vi "nanocal_raw_file_manage_V1.vi"(7 "action":T2, 10 "list of lines IN":string[](array[string]), 11 "header IN":string) -> (0 "z (K/W)  OUT":cdb[](array[numeric]), 1 "f (Hz) OUT":dbl[](array[numeric]), 3 "header OUT":string)   [LabVIEW 2021]
uses:
  nanocal_raw_file_manage_fieldname_V1.ctl
  nanocal_raw_file_manage_action_V1.ctl
panel:
  out "test IN":string[][](array[string])
  out "Map":map{T1, i32}(c390)
  in  "Text Ring":u16(ring) items=["Time (s)", "Datapoint index", "Datapoint time (s)", "PHs (W)", "PHr (W)", "Ps,dc (W)", "Pr,dc (W)", "PHs,dc (W)", "PHr,dc (W)", "Ps,ac (W)", "Pr,ac (W)", "PHs/PHr", "Poffs (W)", "Ps total (W)", "Pr total (W)", "Ps-Pr total (W)", "Ps,offs (W)", "Ps,cond (W)", "Ps,net (W)", "Cs (J/K)", "Ks (W/K)", "Cr (J/K)", "Kr (W/K)", "Cdiff (J/K)", "Cs-Cr (J/K)", "Cdiff old style (J/K)", "Cr from S,diff (J/K)", "Cs from dT/dt (J/K)", "Ks,nom (W/K)", "Cs/T (J/K^2)", "Cr/T (J/K^2)", "Cdiff/T (J/K^2)", "(Cs-Cr)/T (J/K^2)", "Cdiff/T old style (J/K^2)", "Cr/T from S,diff (J/K^2)", "Ts (K)", "Tr (K)", "Tdiff from Rs,Rr", "Tdiff from Udiff (K)", "Ts,ac (K)", "Tr,ac (K)", "Tdiff,ac (K)", "Ts,ac driftcorr (K)", "Tr,ac driftcorr (K)", "Tr,ac from Ts,diff,ac (K)", "T target (K)", "Ts^2 (K^2)", "Tr^2 (K^2)", "Tcos/(P/K)", "Tsin/(P/K)", "H (T)", "T probe (K)", "Polar angle (deg)", "Azimuthal angle (deg)", "RHs (ohm)", "RHr (ohm)", "Rs (ohm)", "Rr (ohm)", "RHs,dc (ohm)", "RHr,dc (ohm)", "Rs,ac (ohm)", "Rr,ac (ohm)", "Roffs (ohm)", "f (Hz)", "f therm (Hz)", "omega (rad/s)", "Tan Phi S/diff", "Sin Phi", "Cos Phi", "f mix (Hz)", "tau (s)", "Phi Is (deg)", "Phi Us (deg)", "Phi Ir (deg)", "Phi Ur (deg)", "Phi Udiff (deg)", "Phi IHs (deg)", "Phi UHs (deg)", "Phi IHr (deg)", "Phi UHr (deg)", "Phi R from S,diff (deg)", "Phi Is 1st (deg)", "Phi Us 1st (deg)", "Phi Ir 1st (deg)", "Phi Ur 1st (deg)", "Phi Udiff 1st (deg)", "Phi Udiff, raw (deg)", "S phase (deg)", "R phase (deg)", "Diff phase (deg)", "Is,dc (A)", "Ir,dc (A)", "Us,dc (V)", "Ur,dc (V)", "Udiff,dc (V)", "IHs dc (A)", "UHs dc (V)", "IHr dc (A)", "UHr dc (V)", "Uoffs dc (V)", "Ioffs dc (A)", "Is,ac 1st (A)", "Ir,ac 1st (A)", "Us,ac 1st (V)", "Ur,ac 1st (V)", "Udiff,ac 1st (V)", "IHs (A)", "UHs (V)", "IHr (A)", "UHr (V)", "Is,ac (A)", "Ir,ac (A)", "Us,ac (V)", "Ur,ac (V)", "Udiff,ac (V)", "S out phase (deg)", "R out phase (deg)", "Hs ac out (Vrms)", "Hr ac out (Vrms)", "S Therm dc out (V)", "R Therm dc out (V)", "S Therm ac out (Vrms)", "R Therm ac out (Vrms)", "Offset dc out (V)", "Hs dc out (V)", "Hr dc out (V)", "Offset ac out (Vrms)", "1+Rs/RIs factor", "1+RIs/Rs factor", "Rs,scaled (ohm)", "Rr,scaled (ohm)", "R lead S (ohm)", "R lead R (ohm)", "|dlnR/dlnT| S", "|dlnR/dlnT| R", "dTs/dt (mK/s)", "dTr/dt (mK/s)", "Test"]
  in  "field names":T1
  out "Array":string[][](array[string])
  in  "String names":string
  in  "String numbers":string
  # "(* {62, (* Phs*) 4,(*Tac*)40, (*phase*)86} -- old file structure*)\n\na2 = rawdata[name]  // \n\n   map2[ {2 (* current to power*)   #[[62]],\n (* use Ts,ac   *) #[[40]]/#[[4]] Cos[ #[[86]]  Pi /180],  \n                            #[[40]]/#[[4]] Sin[ #[[86]]  Pi /180] \n\n} &] ;"
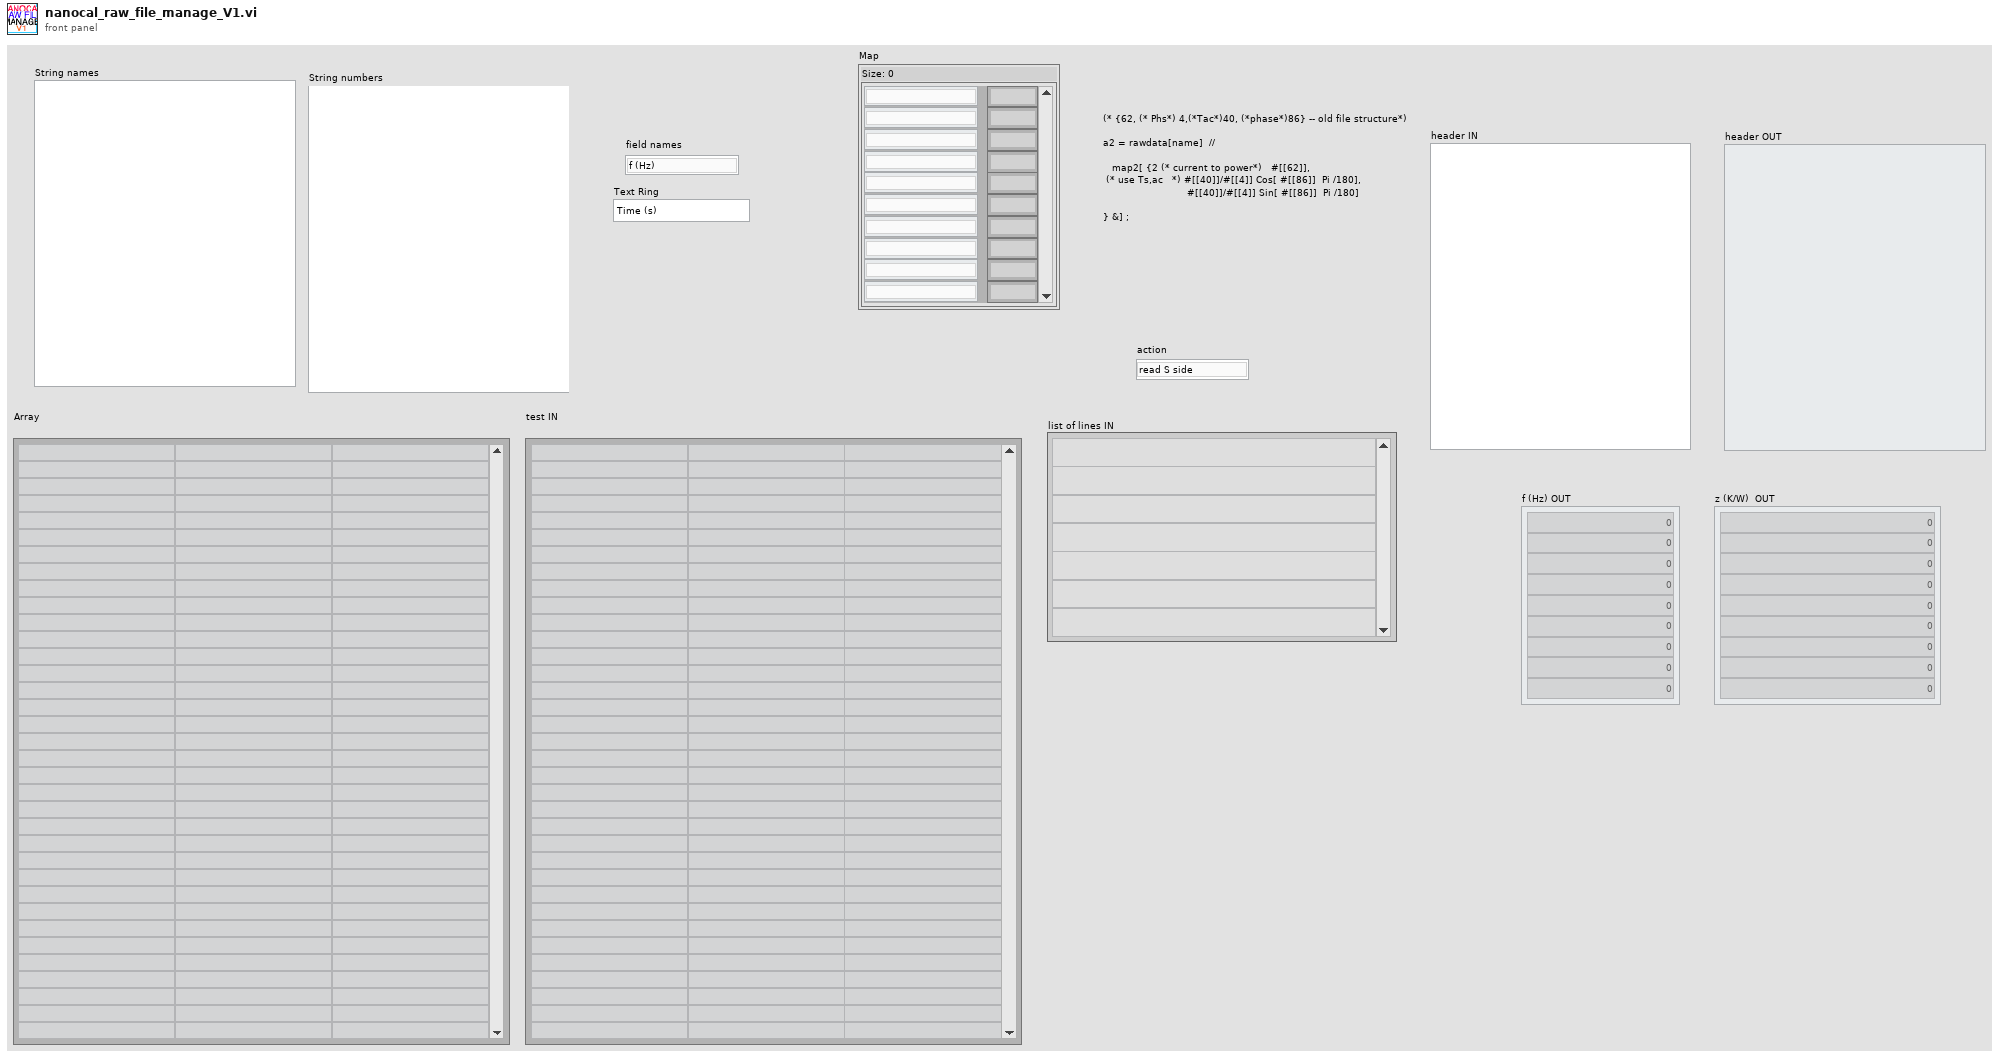
[diagram p1: front panel]
types:
  T1 = typedef "nanocal_raw_file_manage_fieldname_V1.ctl" = enum16{"f (Hz)", "S phase (deg)", "R phase (deg)", "Ts,ac (K)", "Tr,ac (K)", "PHs (W)", "PHr (W)", "Time (s)", "Tdiff,ac (K)", "Ts (K)", "Tr (K)"}
  T2 = typedef "nanocal_raw_file_manage_action_V1.ctl" = enum16{"read S side", "read R side", "read meta", "read_names"}
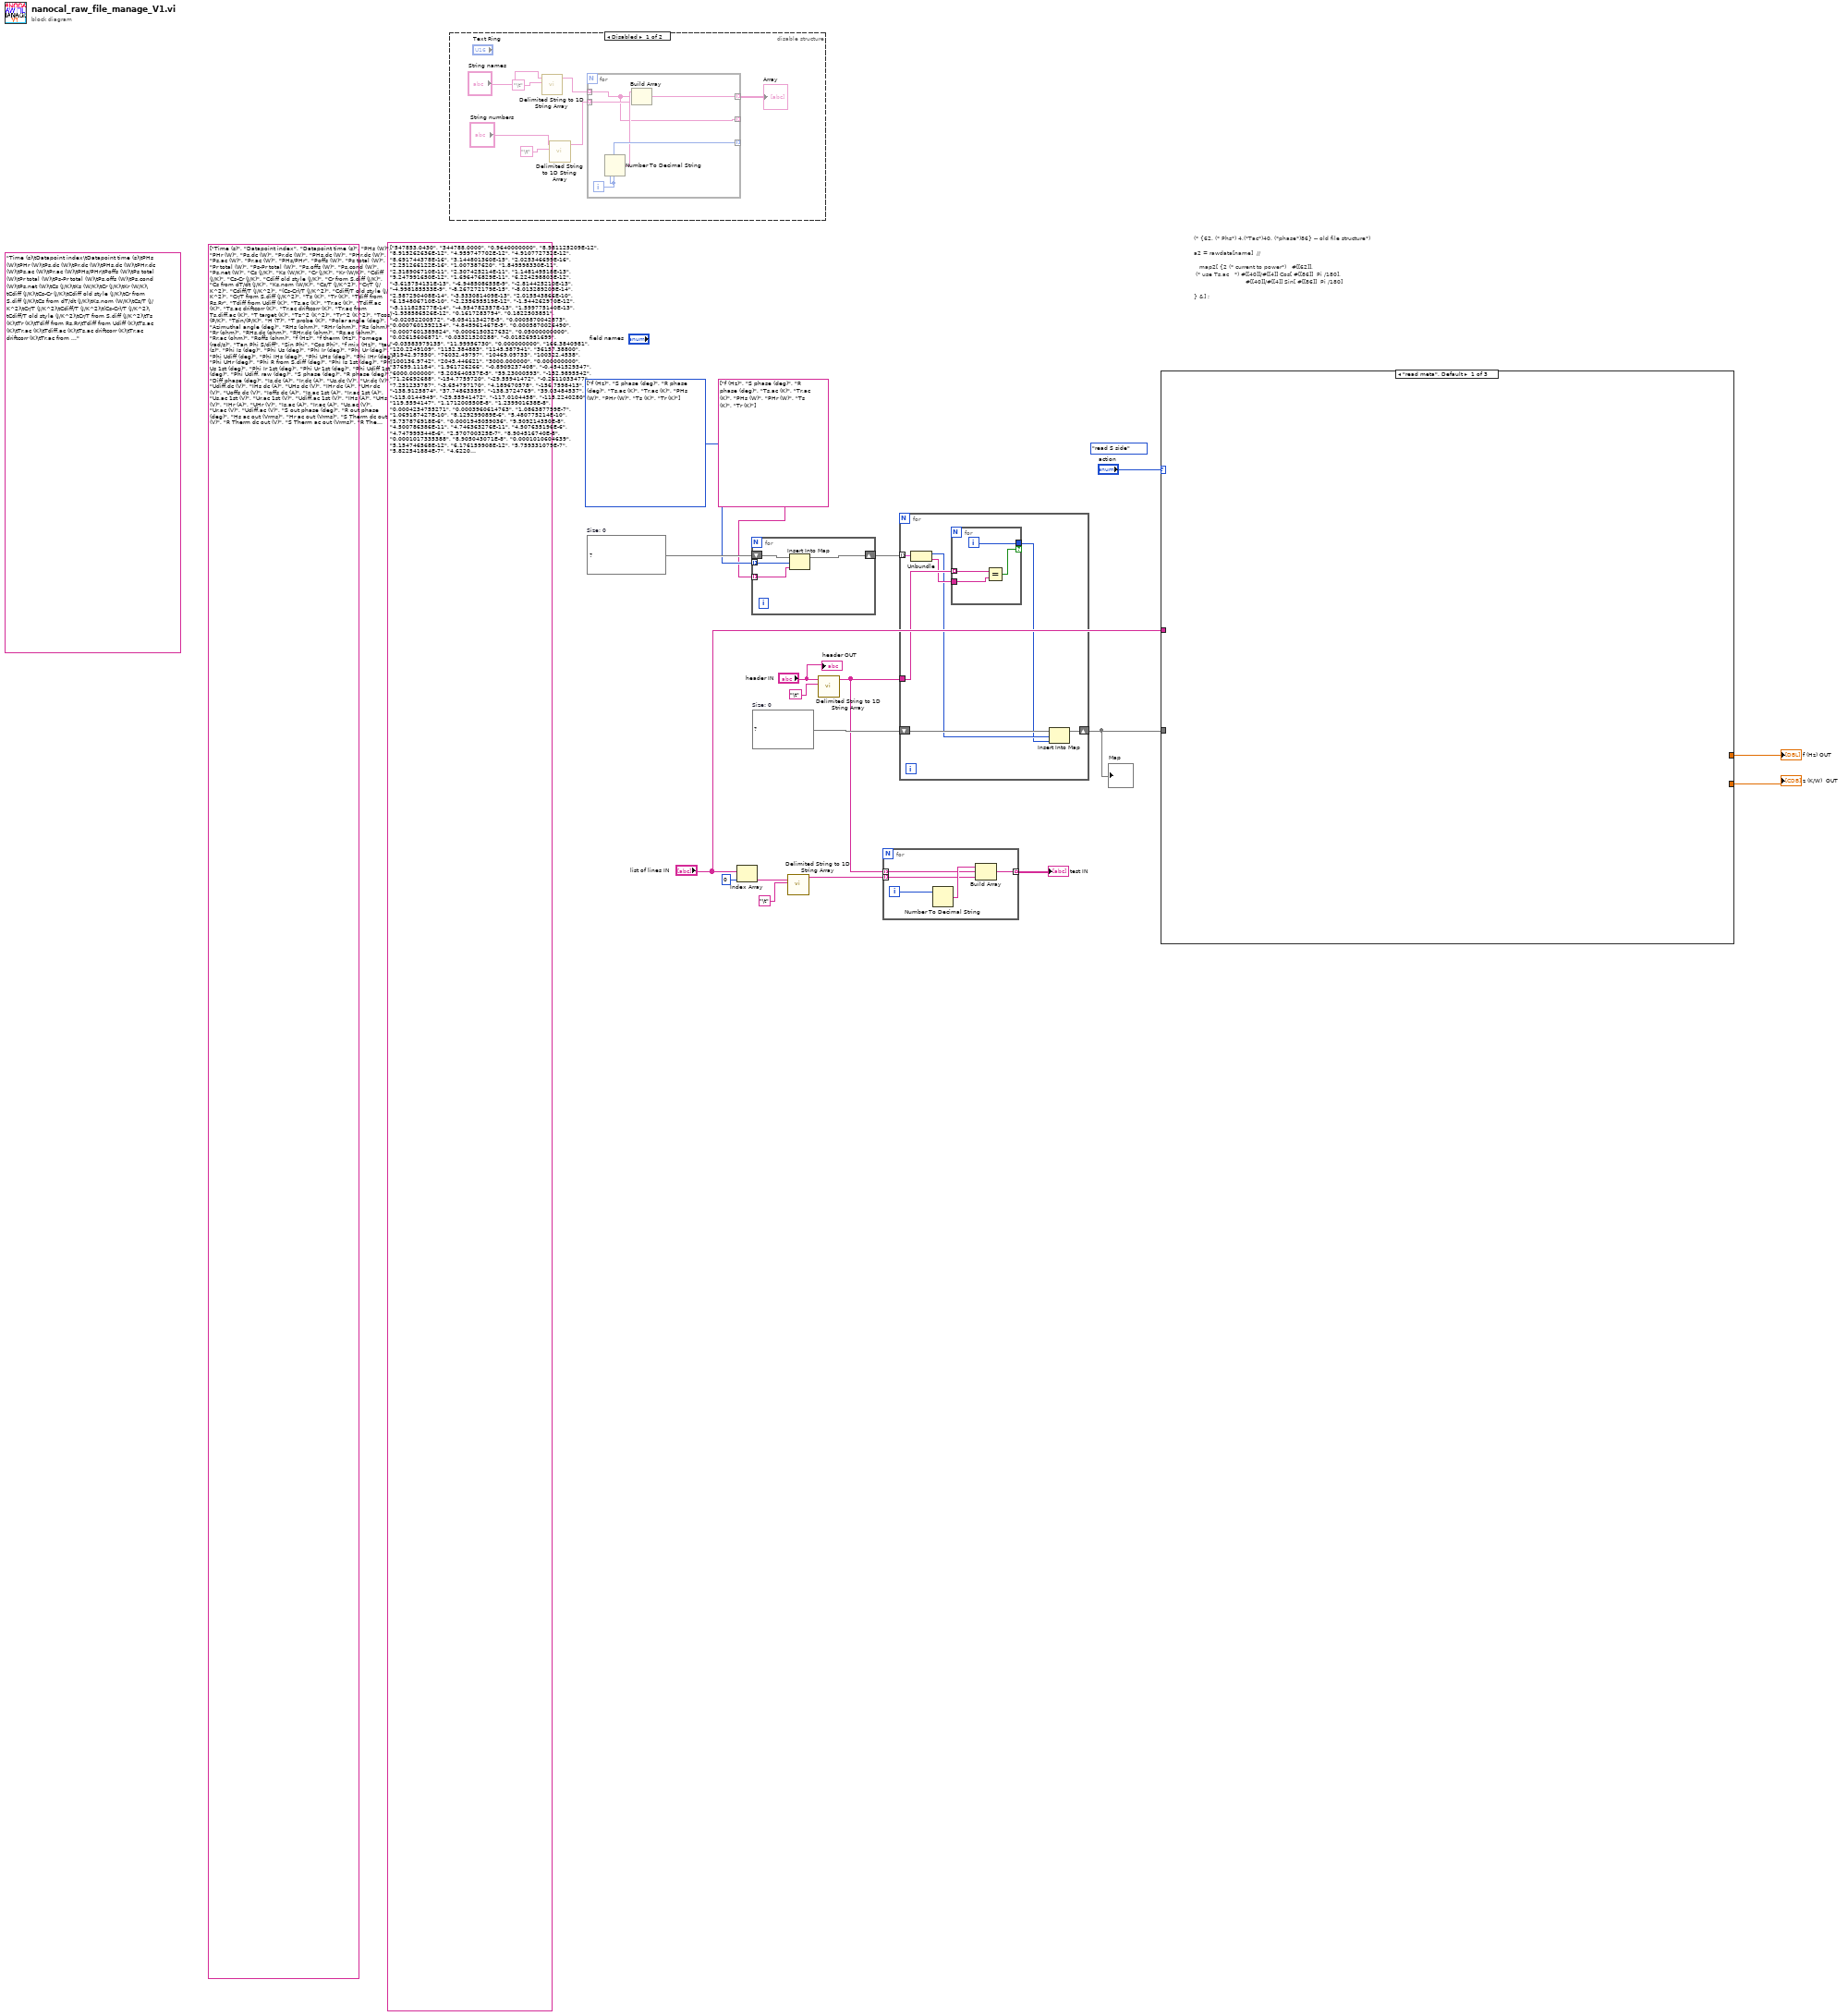
[diagram p0: block diagram]
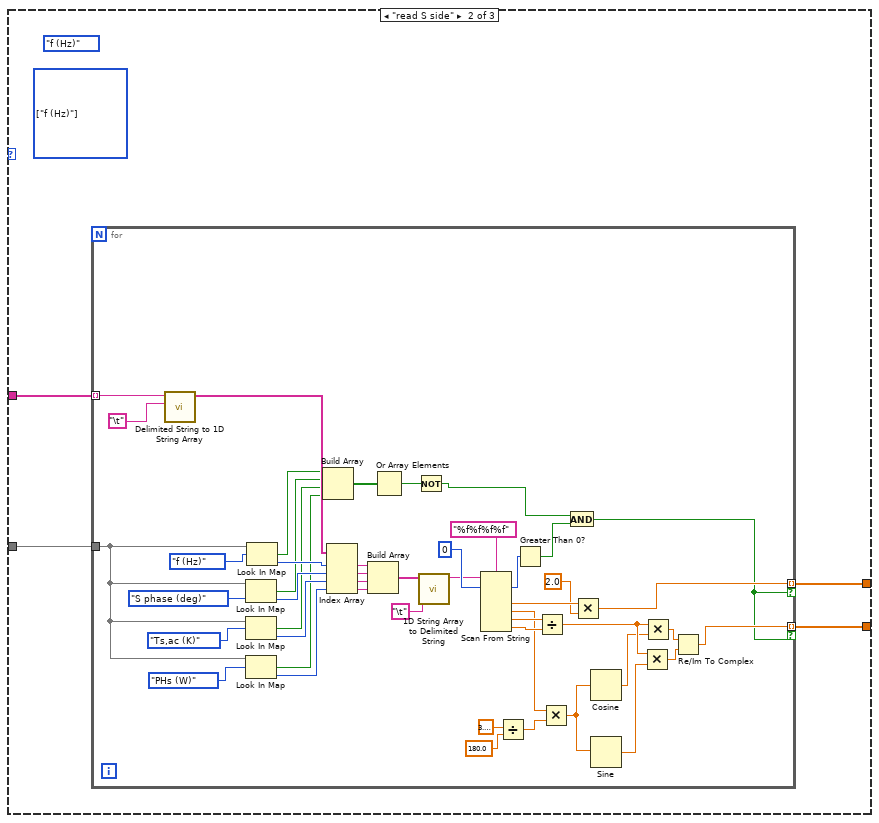
[diagram p3: hidden frame]
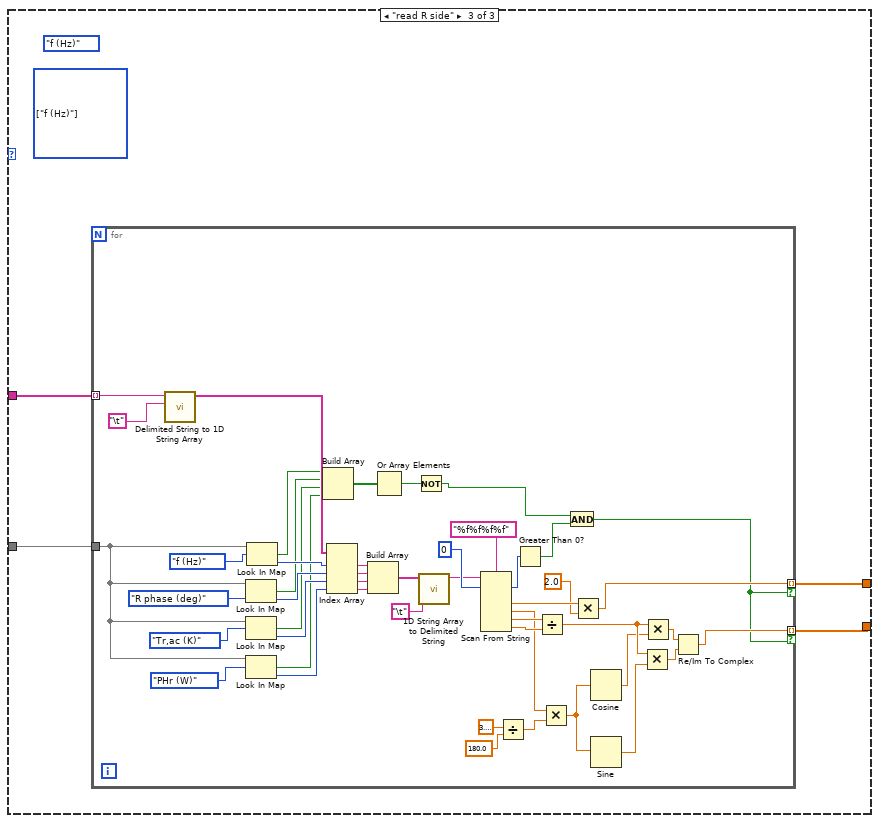
[diagram p4: hidden frame]
diagram:
  w13 = map{T1, i32} {}  # Size: 0
  w17 = map{T1, string} {}  # Size: 0
  w16 = T1[] [enum."f (Hz)", enum."S phase (deg)", enum."R phase (deg)", enum."Ts,ac (K)", enum."Tr,ac (K)", enum."PHs (W)", enum."PHr (W)", enum."Ts (K)", enum."Tr (K)"] items=["f (Hz)", "S phase (deg)", "R phase (deg)", "Ts,ac (K)", "Tr,ac (K)", "PHs (W)", "PHr (W)", "Time (s)", "Tdiff,ac (K)", "Ts (K)", "Tr (K)"]
  (unwired) nanocal_raw_file_manage_action_V1."read S side" ("Enum")
  (unwired) string[] ["547853.0430", "344788.0000", "0.9640000000", "8.981125209E-12", "8.915262636E-12", "4.959747702E-12", "4.910772732E-12", "8.691744378E-16", "3.144801360E-15", "2.025346699E-16", "2.251266122E-16", "1.007387620", "1.849598330E-11", "2.318906710E-11", "2.307425214E-11", "1.148149518E-13", "9.247991650E-12", "1.696476829E-11", "6.224298803E-12", "-3.615754131E-13", "-6.948508655E-9", "-2.814425210E-13", "-4.998185533E-9", "-8.267272179E-15", "-8.013289209E-14", "2.587290408E-14", "-3.533081409E-13", "2.015543866E-10", "6.154806710E-10", "-2.235695519E-12", "-1.544262970E-12", "-5.111825277E-14", "-4.954782357E-13", "1.599775140E-13", "-1.938586526E-12", "0.1617283794", "0.1822503851", "-0.02052200572", "-8.054113427E-5", "0.0005870042873", "0.0007601392134", "4.845961467E-5", "0.0005870026490", "0.0007601389824", "0.0006150327632", "0.05000000000", "0.02615606871", "0.03321520288", "-0.01826951699", "-0.03583979135", "11.99956730", "0.000000000", "166.3840981", "120.2249109", "1152.384883", "1145.587941", "36157.38800", "31942.97550", "76032.49797", "10469.09733", "100322.4538", "100136.9742", "2045.446621", "3000.000000", "0.000000000", "37699.11184", "1.961726266", "-0.8909237408", "-0.4541529347", "6000.000000", "5.203640537E-5", "59.23000593", "-152.9895542", "71.26692688", "-154.7759720", "-29.55941472", "-0.2611033477", "7.251233787", "-3.654797170", "4.189670578", "-156.7598413", "-138.9125874", "37.74863355", "-138.3724769", "39.03484537", "-115.0144949", "-29.55941472", "-117.0104458", "-115.2240280", "119.5594147", "1.171200550E-8", "1.239901638E-8", "0.0004234755271", "0.0003960614763", "1.086387799E-7", "1.069187427E-10", "8.129299089E-6", "5.480775214E-10", "5.737876918E-6", "0.0001945059036", "9.509214350E-8", "4.500786386E-11", "4.746363276E-11", "4.507635196E-6", "4.747999344E-6", "2.570700325E-7", "8.904516740E-8", "0.0001017335388", "8.905043071E-8", "0.0001010604639", "5.154746568E-12", "6.176159908E-12", "5.759331079E-7", "5.822541884E-7", "4.622022938E-8", "0.000000000", "0.000000000", "0.009030217479", "0.009030217479", "0.001382604241", "0.001487392001", "0.000000000", "0.000000000", "0.009530331008", "0.000000000", "0.000000000", "0.000000000", "1.361573880", "3.765686503", "36157.38800", "31942.97550", "-18107.21790", "-11982.49189", "0.7014008160", "0.6673683771", "0.03088148519", "0.004354902059", "1.234560000"] ("string array")
  (unwired) "Time (s)\tDatapoint index\tDatapoint time (s)\tPHs (W)\tPHr (W)\tPs,dc (W)\tPr,dc (W)\tPHs,dc (W)\tPHr,dc (W)\tPs,ac (W)\tPr,ac (W)\tPHs/PHr\tPoffs (W)\tPs total (W)\tPr total (W)\tPs-Pr total (W)\tPs,offs (W)\tPs,cond (W)\tPs,net (W)\tCs (J/K)\tKs (W/K)\tCr (J/K)\tKr (W/K)\tCdiff (J/K)\tCs-Cr (J/K)\tCdiff old style (J/K)\tCr from S,diff (J/K)\tCs from dT/dt (J/K)\tKs,nom (W/K)\tCs/T (J/K^2)\tCr/T (J/K^2)\tCdiff/T (J/K^2)\t(Cs-Cr)/T (J/K^2)\tCdiff/T old style (J/K^2)\tCr/T from S,diff (J/K^2)\tTs (K)\tTr (K)\tTdiff from Rs,Rr\tTdiff from Udiff (K)\tTs,ac (K)\tTr,ac (K)\tTdiff,ac (K)\tTs,ac driftcorr (K)\tTr,ac driftcorr (K)\tTr,ac from Ts,diff,ac (K)\tT target (K)\tTs^2 (K^2)\tTr^2 (K^2)\tTcos/(P/K)\tTsin/(P/K)\tH (T)\tT probe (K)\tPolar angle (deg)\tAzimuthal angle (deg)\tRHs (ohm)\tRHr (ohm)\tRs (ohm)\tRr (ohm)\tRHs,dc (ohm)\tRHr,dc (ohm)\tRs,ac (ohm)\tRr,ac (ohm)\tRoffs (ohm)\tf (Hz)\tf therm (Hz)\tomega (rad/s)\tTan Phi S/diff\tSin Phi\tCos Phi\tf mix (Hz)\ttau (s)\tPhi Is (deg)\tPhi Us (deg)\tPhi Ir (deg)\tPhi Ur (deg)\tPhi Udiff (deg)\tPhi IHs (deg)\tPhi UHs (deg)\tPhi IHr (deg)\tPhi UHr (deg)\tPhi R from S,diff (deg)\tPhi Is 1st (deg)\tPhi Us 1st (deg)\tPhi Ir 1st (deg)\tPhi Ur 1st (deg)\tPhi Udiff 1st (deg)\tPhi Udiff, raw (deg)\tS phase (deg)\tR phase (deg)\tDiff phase (deg)\tIs,dc (A)\tIr,dc (A)\tUs,dc (V)\tUr,dc (V)\tUdiff,dc (V)\tIHs dc (A)\tUHs dc (V)\tIHr dc (A)\tUHr dc (V)\tUoffs dc (V)\tIoffs dc (A)\tIs,ac 1st (A)\tIr,ac 1st (A)\tUs,ac 1st (V)\tUr,ac 1st (V)\tUdiff,ac 1st (V)\tIHs (A)\tUHs (V)\tIHr (A)\tUHr (V)\tIs,ac (A)\tIr,ac (A)\tUs,ac (V)\tUr,ac (V)\tUdiff,ac (V)\tS out phase (deg)\tR out phase (deg)\tHs ac out (Vrms)\tHr ac out (Vrms)\tS Therm dc out (V)\tR Therm dc out (V)\tS Therm ac out (Vrms)\tR Therm ac out (Vrms)\tOffset dc out (V)\tHs dc out (V)\tHr dc out (V)\tOffset ac out (Vrms)\t1+Rs/RIs factor\t1+RIs/Rs factor\tRs,scaled (ohm)\tRr,scaled (ohm)\tR lead S (ohm)\tR lead R (ohm)\t|dlnR/dlnT| S\t|dlnR/dlnT| R\tdTs/dt (mK/s)\tdTr/dt (mK/s)\tTest\t\n" ("String")
  (unwired) string[] ["Time (s)", "Datapoint index", "Datapoint time (s)", "PHs (W)", "PHr (W)", "Ps,dc (W)", "Pr,dc (W)", "PHs,dc (W)", "PHr,dc (W)", "Ps,ac (W)", "Pr,ac (W)", "PHs/PHr", "Poffs (W)", "Ps total (W)", "Pr total (W)", "Ps-Pr total (W)", "Ps,offs (W)", "Ps,cond (W)", "Ps,net (W)", "Cs (J/K)", "Ks (W/K)", "Cr (J/K)", "Kr (W/K)", "Cdiff (J/K)", "Cs-Cr (J/K)", "Cdiff old style (J/K)", "Cr from S,diff (J/K)", "Cs from dT/dt (J/K)", "Ks,nom (W/K)", "Cs/T (J/K^2)", "Cr/T (J/K^2)", "Cdiff/T (J/K^2)", "(Cs-Cr)/T (J/K^2)", "Cdiff/T old style (J/K^2)", "Cr/T from S,diff (J/K^2)", "Ts (K)", "Tr (K)", "Tdiff from Rs,Rr", "Tdiff from Udiff (K)", "Ts,ac (K)", "Tr,ac (K)", "Tdiff,ac (K)", "Ts,ac driftcorr (K)", "Tr,ac driftcorr (K)", "Tr,ac from Ts,diff,ac (K)", "T target (K)", "Ts^2 (K^2)", "Tr^2 (K^2)", "Tcos/(P/K)", "Tsin/(P/K)", "H (T)", "T probe (K)", "Polar angle (deg)", "Azimuthal angle (deg)", "RHs (ohm)", "RHr (ohm)", "Rs (ohm)", "Rr (ohm)", "RHs,dc (ohm)", "RHr,dc (ohm)", "Rs,ac (ohm)", "Rr,ac (ohm)", "Roffs (ohm)", "f (Hz)", "f therm (Hz)", "omega (rad/s)", "Tan Phi S/diff", "Sin Phi", "Cos Phi", "f mix (Hz)", "tau (s)", "Phi Is (deg)", "Phi Us (deg)", "Phi Ir (deg)", "Phi Ur (deg)", "Phi Udiff (deg)", "Phi IHs (deg)", "Phi UHs (deg)", "Phi IHr (deg)", "Phi UHr (deg)", "Phi R from S,diff (deg)", "Phi Is 1st (deg)", "Phi Us 1st (deg)", "Phi Ir 1st (deg)", "Phi Ur 1st (deg)", "Phi Udiff 1st (deg)", "Phi Udiff, raw (deg)", "S phase (deg)", "R phase (deg)", "Diff phase (deg)", "Is,dc (A)", "Ir,dc (A)", "Us,dc (V)", "Ur,dc (V)", "Udiff,dc (V)", "IHs dc (A)", "UHs dc (V)", "IHr dc (A)", "UHr dc (V)", "Uoffs dc (V)", "Ioffs dc (A)", "Is,ac 1st (A)", "Ir,ac 1st (A)", "Us,ac 1st (V)", "Ur,ac 1st (V)", "Udiff,ac 1st (V)", "IHs (A)", "UHs (V)", "IHr (A)", "UHr (V)", "Is,ac (A)", "Ir,ac (A)", "Us,ac (V)", "Ur,ac (V)", "Udiff,ac (V)", "S out phase (deg)", "R out phase (deg)", "Hs ac out (Vrms)", "Hr ac out (Vrms)", "S Therm dc out (V)", "R Therm dc out (V)", "S Therm ac out (Vrms)", "R Therm ac out (Vrms)", "Offset dc out (V)", "Hs dc out (V)", "Hr dc out (V)", "Offset ac out (Vrms)", "1+Rs/RIs factor", "1+RIs/Rs factor", "Rs,scaled (ohm)", "Rr,scaled (ohm)", "R lead S (ohm)", "R lead R (ohm)", "|dlnR/dlnT| S", "|dlnR/dlnT| R", "dTs/dt (mK/s)", "dTr/dt (mK/s)", "Test", ""] ("string array")
  # "(* {62, (* Phs*) 4,(*Tac*)40, (*phase*)86} -- old file structure*)\n\na2 = rawdata[name]  // \n\n   map2[ {2 (* current to power*)   #[[62]],\n (* use Ts,ac   *) #[[40]]/#[[4]] Cos[ #[[86]]  Pi /180],  \n                            #[[40]]/#[[4]] Sin[ #[[86]]  Pi /180] \n\n} &] ;"
  n1 = disable-structure shown="Disabled" {
    frame Disabled {
      n2 = call <vilib>:"Delimited String to 1D String Array.vi"("delimiter"="\t", "delimited string"="String names") -> ("string array"=w19:string[])  [unwired: 9 in]
      n3 = call <vilib>:"Delimited String to 1D String Array.vi"("delimiter"="\t", "delimited string"="String numbers") -> ("string array"=w23:string[])  [unwired: 9 in]
      n4 = for {
        tunnel: w23 -> [w27] mode=indexing
        tunnel: [w28] -> w22 mode=indexing
        tunnel: [w30] -> _ mode=indexing
        tunnel: w19 -> [w26] mode=indexing
        tunnel: [w26] -> _ mode=indexing
        i -> [w30]
        n5 = Number To Decimal String(number=w30) -> (decimal integer string=w29:string)  [unwired: 1 in]
        n6 = Build Array(w29, w26, w27) -> (w28:string[])
      }
      "Array" <- w22
    }
    frame Enabled {
    }
  }
  n7 = Index Array(array="list of lines IN", index=0 ("index (row)")) -> (element=w9:string)
  n8 = for {
    shift-right: [w33] -> w12
    shift-left: w17 -> [w34]
    tunnel: w16 -> [w32] mode=indexing
    tunnel: string[] ["f (Hz)", "S phase (deg)", "R phase (deg)", "Ts,ac (K)", "Tr,ac (K)", "PHs (W)", "PHr (W)", "Ts (K)", "Tr (K)"] -> [w31] mode=indexing
    n9 = Insert Into Map(map in=w34, key=w32, value=w31) -> (map out=w33:map{T1, string})  [unwired: 2 out]
  }
  n10 = call <vilib>:"Delimited String to 1D String Array.vi"("delimiter"="\t", "delimited string"=w9) -> ("string array"=w7:string[])  [unwired: 9 in]
  n11 = call <vilib>:"Delimited String to 1D String Array.vi"("delimiter"="\t", "delimited string"="header IN") -> ("string array"=w11:string[])  [unwired: 9 in]
  n12 = for {
    tunnel: w7 -> [w36] mode=indexing
    tunnel: [w37] -> w6 mode=indexing
    tunnel: w11 -> [w35] mode=indexing
    i -> [w39]
    n13 = Number To Decimal String(number=w39) -> (decimal integer string=w38:string)  [unwired: 1 in]
    n14 = Build Array(w38, w35, w36) -> (w37:string[])
  }
  "test IN" <- w6
  n15 = for {
    shift-right: [w45] -> w5
    shift-left: w13 -> [w46]
    tunnel: w11 -> [w44]
    tunnel: w12 -> [w43] mode=indexing
    n16 = Unbundle(w43) -> ("field names"=w41:T1, w42:string)
    n17 = for {
      tunnel: w44 -> [w50] mode=indexing
      tunnel: w42 -> [w49]
      tunnel: [w48] -> w40 if=w47
      i -> [w48]
      n18 = Equal?(x=w50, y=w49) -> (x = y?=w47:bool)
    }
    n19 = Insert Into Map(map in=w46, key=w41, value=w40) -> (map out=w45:map{T1, i32})  [unwired: 2 out]
  }
  "Map" <- w5
  n20 = case shown="\"read meta\", Default" "action" {
    tunnel: w5 -> [_ w53 w104]
    tunnel: "list of lines IN" -> [_ w54 w105]
    tunnel: [_ w52 w103] -> w2
    tunnel: [_ w51 w102] -> w1
    frame "read meta", Default {
    }
    frame "read S side" {
      (unwired) T1[] [enum."f (Hz)"] items=["f (Hz)", "S phase (deg)", "R phase (deg)", "Ts,ac (K)", "Tr,ac (K)", "PHs (W)", "PHr (W)", "Time (s)", "Tdiff,ac (K)", "Ts (K)", "Tr (K)"]
      (unwired) nanocal_raw_file_manage_fieldname_V1."f (Hz)" ("field names")
      n21 = for {
        tunnel: w54 -> [w101] mode=indexing
        tunnel: w53 -> [w97]
        tunnel: [w57] -> w52 mode=indexing if=w55
        tunnel: [w56] -> w51 mode=indexing if=w55
        n22 = call <vilib>:"Delimited String to 1D String Array.vi"("delimiter"="\t", "delimited string"=w101) -> ("string array"=w94:string[])  [unwired: 9 in]
        n23 = Look In Map(map=w97, key=nanocal_raw_file_manage_fieldname_V1."S phase (deg)" ("field names")) -> (key not found?=w80:bool, value=w92:i32)  [unwired: 1 in]
        n24 = Look In Map(map=w97, key=nanocal_raw_file_manage_fieldname_V1."Ts,ac (K)" ("field names")) -> (key not found?=w79:bool, value=w91:i32)  [unwired: 1 in]
        n25 = Look In Map(map=w97, key=nanocal_raw_file_manage_fieldname_V1."PHs (W)" ("field names")) -> (key not found?=w78:bool, value=w90:i32)  [unwired: 1 in]
        n26 = Look In Map(map=w97, key=nanocal_raw_file_manage_fieldname_V1."f (Hz)" ("field names")) -> (key not found?=w81:bool, value=w93:i32)  [unwired: 1 in]
        n27 = Build Array(w81, w80, w79, w78) -> (w61:bool[])
        n28 = Index Array(array=w94, index #1=w93, index #2=w92, index #3=w91, index #4=w90) -> (element #1=w86:string, element #2=w85:string, element #3=w84:string, element #4=w83:string)
        n29 = Build Array(w86, w85, w84, w83) -> (w77:string[])
        n30 = Or Array Elements(Boolean array=w61) -> (logical OR=w60:bool)
        n31 = Not(x=w60) -> (.not. x?=w58:bool)
        n32 = call <vilib>:"1D String Array to Delimited String.vi"("delimiter"="\t", "string array"=w77) -> ("delimited string"=w75:string)  [unwired: 9 in]
        n33 = Scan From String(format string="%f%f%f%f", input string=w75, initial scan location=u32 0) -> (offset past scan=w87:u32, output 1=w82:dbl, output 2=w68:dbl, output 3=w73:dbl, output 4=w72:dbl)  [unwired: 5 in, 2 out]
        n34 = Divide(x=3.141592653589793, y=180.0) -> (x/y=w69:dbl)
        n35 = Greater Than 0?(x=w87) -> (x > 0?=w59:bool)
        n36 = Divide(x=w73, y=w72) -> (x/y=w66:dbl)
        n37 = Multiply(x=w68, y=w69) -> (x*y=w64:dbl)
        n38 = And(x=w58, y=w59) -> (x .and. y?=w55:bool)
        n39 = Multiply(x=w82, y=2.0) -> (x*y=w57:dbl)
        n40 = Cosine(x=w64) -> (cos(x)=w63:dbl)
        n41 = Sine(x=w64) -> (sin(x)=w62:dbl)
        n42 = Multiply(x=w66, y=w62) -> (x*y=w65:dbl)
        n43 = Multiply(x=w66, y=w63) -> (x*y=w67:dbl)
        n44 = Re/Im To Complex(1:w65, 2:w67) -> (0:w56:cdb)
      }
    }
    frame "read R side" {
      (unwired) T1[] [enum."f (Hz)"] items=["f (Hz)", "S phase (deg)", "R phase (deg)", "Ts,ac (K)", "Tr,ac (K)", "PHs (W)", "PHr (W)", "Time (s)", "Tdiff,ac (K)", "Ts (K)", "Tr (K)"]
      (unwired) nanocal_raw_file_manage_fieldname_V1."f (Hz)" ("field names")
      n45 = for {
        tunnel: w105 -> [w152] mode=indexing
        tunnel: w104 -> [w148]
        tunnel: [w108] -> w103 mode=indexing if=w106
        tunnel: [w107] -> w102 mode=indexing if=w106
        n46 = call <vilib>:"Delimited String to 1D String Array.vi"("delimiter"="\t", "delimited string"=w152) -> ("string array"=w145:string[])  [unwired: 9 in]
        n47 = Look In Map(map=w148, key=nanocal_raw_file_manage_fieldname_V1."R phase (deg)" ("field names")) -> (key not found?=w131:bool, value=w143:i32)  [unwired: 1 in]
        n48 = Look In Map(map=w148, key=nanocal_raw_file_manage_fieldname_V1."Tr,ac (K)" ("field names")) -> (key not found?=w130:bool, value=w142:i32)  [unwired: 1 in]
        n49 = Look In Map(map=w148, key=nanocal_raw_file_manage_fieldname_V1."PHr (W)" ("field names")) -> (key not found?=w129:bool, value=w141:i32)  [unwired: 1 in]
        n50 = Look In Map(map=w148, key=nanocal_raw_file_manage_fieldname_V1."f (Hz)" ("field names")) -> (key not found?=w132:bool, value=w144:i32)  [unwired: 1 in]
        n51 = Build Array(w132, w131, w130, w129) -> (w112:bool[])
        n52 = Index Array(array=w145, index #1=w144, index #2=w143, index #3=w142, index #4=w141) -> (element #1=w137:string, element #2=w136:string, element #3=w135:string, element #4=w134:string)
        n53 = Build Array(w137, w136, w135, w134) -> (w128:string[])
        n54 = Or Array Elements(Boolean array=w112) -> (logical OR=w111:bool)
        n55 = Not(x=w111) -> (.not. x?=w109:bool)
        n56 = call <vilib>:"1D String Array to Delimited String.vi"("delimiter"="\t", "string array"=w128) -> ("delimited string"=w126:string)  [unwired: 9 in]
        n57 = Scan From String(format string="%f%f%f%f", input string=w126, initial scan location=u32 0) -> (offset past scan=w138:u32, output 1=w133:dbl, output 2=w119:dbl, output 3=w124:dbl, output 4=w123:dbl)  [unwired: 5 in, 2 out]
        n58 = Divide(x=3.141592653589793, y=180.0) -> (x/y=w120:dbl)
        n59 = Greater Than 0?(x=w138) -> (x > 0?=w110:bool)
        n60 = Divide(x=w124, y=w123) -> (x/y=w117:dbl)
        n61 = Multiply(x=w119, y=w120) -> (x*y=w115:dbl)
        n62 = And(x=w109, y=w110) -> (x .and. y?=w106:bool)
        n63 = Multiply(x=w133, y=2.0) -> (x*y=w108:dbl)
        n64 = Cosine(x=w115) -> (cos(x)=w114:dbl)
        n65 = Sine(x=w115) -> (sin(x)=w113:dbl)
        n66 = Multiply(x=w117, y=w113) -> (x*y=w116:dbl)
        n67 = Multiply(x=w117, y=w114) -> (x*y=w118:dbl)
        n68 = Re/Im To Complex(1:w116, 2:w118) -> (0:w107:cdb)
      }
    }
  }
  "f (Hz) OUT" <- w2
  "z (K/W)  OUT" <- w1
  "header OUT" <- "header IN"
